vi "get Code.vi"(7 "strDate":string, 8 "error in (no error)":errorcluster caption="错误输入（无错误）", 9 "sSN":string, 10 ".NET:EEPromCodeService.ParaClass":T1, 11 "EEPromCodeService 引用句柄":refnum<k24>) -> (0 "error out":errorcluster caption="错误输出", 2 "getCode":string[](array[string]), 3 "EEPromCodeService 引用句柄输出":refnum<k24>)   [LabVIEW 2011]
uses:
  Data/EEPromCodeService.dll
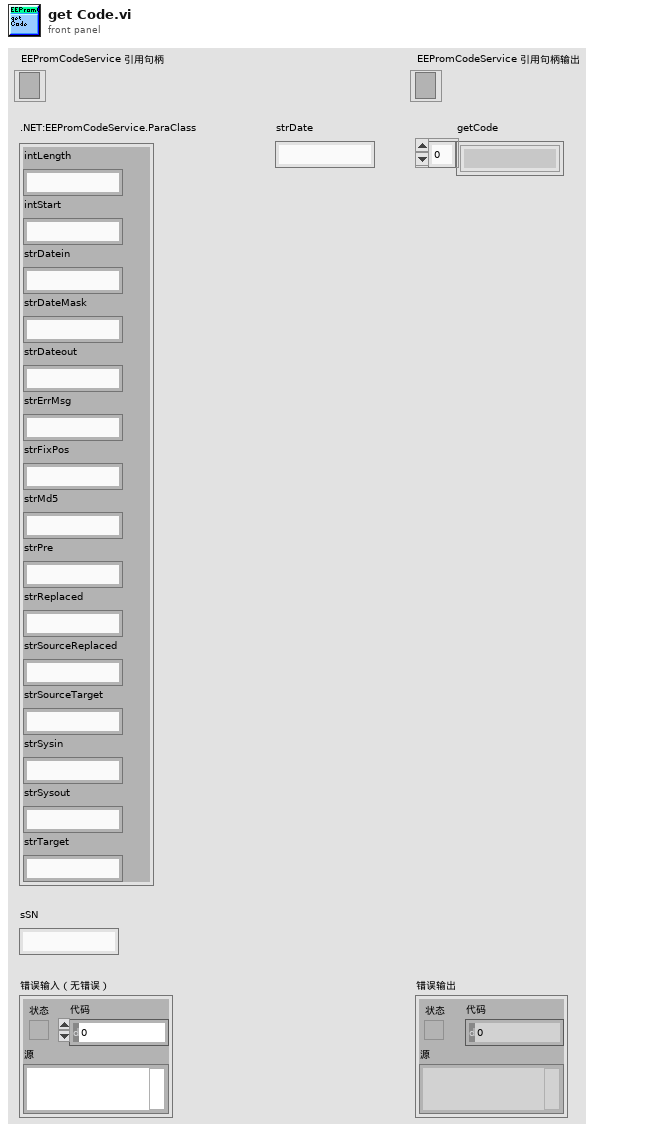
[diagram p1: front panel]
types:
  T1 = cluster{"intLength":string, "intStart":string, "strDatein":string, "strDateMask":string, "strDateout":string, "strErrMsg":string, "strFixPos":string, "strMd5":string, "strPre":string, "strReplaced":string, "strSourceReplaced":string, "strSourceTarget":string, "strSysin":string, "strSysout":string, "strTarget":string}
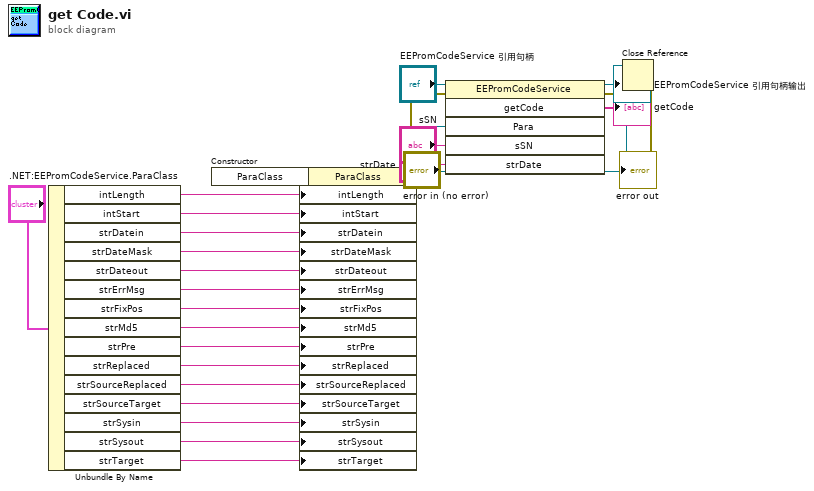
[diagram p0: block diagram]
diagram:
  n1 = Unbundle By Name(".NET:EEPromCodeService.ParaClass") -> ("intLength"=w21:string, "intStart"=w20:string, "strDatein"=w19:string, "strDateMask"=w18:string, "strDateout"=w17:string, "strErrMsg"=w16:string, "strFixPos"=w15:string, "strMd5"=w14:string, "strPre"=w13:string, "strReplaced"=w12:string, "strSourceReplaced"=w11:string, "strSourceTarget"=w10:string, "strSysin"=w9:string, "strSysout"=w8:string, "strTarget"=w7:string)
  n2 = constructor class="ParaClass"(error in="error in (no error)") -> (reference out=w25:refnum<k24>, error out=w24:errorcluster)  [unwired: 2 in, 1 out]
  n3 = property class="ParaClass"(reference=w25, error in=w24, "intLength"=w21, "intStart"=w20, "strDatein"=w19, "strDateMask"=w18, "strDateout"=w17, "strErrMsg"=w16, "strFixPos"=w15, "strMd5"=w14, "strPre"=w13, "strReplaced"=w12, "strSourceReplaced"=w11, "strSourceTarget"=w10, "strSysin"=w9, "strSysout"=w8, "strTarget"=w7) -> (reference out=w23:refnum<k24>, error out=w3:errorcluster)
  n4 = invoke class="EEPromCodeService" method="getCode"(reference="EEPromCodeService 引用句柄", error in=w3, "Para"=w23, "sSN"="sSN", "strDate"="strDate") -> (reference out=→"EEPromCodeService 引用句柄输出":refnum<k24>, error out=w2:errorcluster, "getCode"=→"getCode":string[])  [unwired: 1 in, 3 out]
  n5 = Close Reference(reference=w23, error in (no error)=w2) -> (error out=→"error out":errorcluster)
